vi "DrawTrail.vi"(8 "error in (no error)":errorcluster, 11 "Pong in":refnum<class "Pong.lvclass">) -> (0 "error out":errorcluster, 3 "Pong out":refnum<class "Pong.lvclass">)   [LabVIEW 2019, in "RT_Game.lvlib" / "Pong.lvclass"]
uses:
  Pong.lvclass
  Game/Coordinate.ctl
  Pong.lvclass/Pong.ctl
  PongBall/PongBall.lvclass
  C:/Users/FreshBob/Dropbox/VIs/myRIO_GameConsole/RT/RT_Game/GameObject/GameObject.lvclass
  Globals.vi
  GameObject/GameObject.lvclass
  Game/Game.lvclass
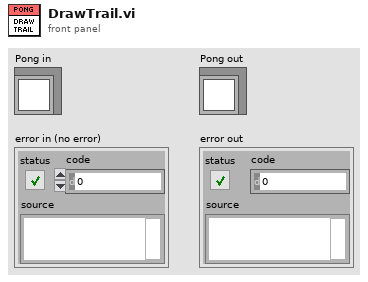
[diagram p1: front panel]
types:
  T1 = typedef "RT_Game.lvlib/Game.lvclass/Coordinate.ctl" = cluster{"x":dbl, "y":dbl}
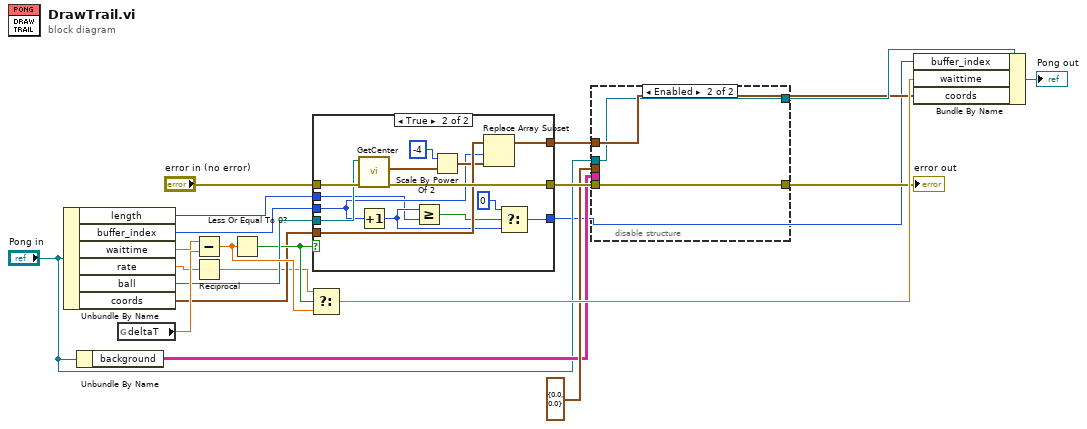
[diagram p0: block diagram]
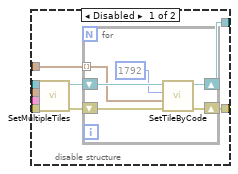
[diagram p2: hidden frame]
diagram:
  n1 = Unbundle By Name("Pong in") -> ("length"=w1:i16, "buffer_index"=w3:i16, "waittime"=w18:dbl, "rate"=w11:dbl, "ball"=w14:refnum<class "PongBall.lvclass">, "coords"=w12:T1[])
  n2 = Unbundle By Name("Pong in") -> ("background"=w5:string[][])
  n3 = global read "Globals.vi" "deltaT"() -> (w17:dbl)
  n4 = Subtract(x=w18, y=w17) -> (x-y=w16:dbl)
  n5 = Reciprocal(x=w11) -> (1/x=w10:dbl)
  n6 = Less Or Equal To 0?(x=w16) -> (x <= 0?=w13:bool)
  n7 = Select(t=w10, s=w13, f=w16) -> (s? t:f=w15:dbl)
  n8 = case shown="True" w13 {
    tunnel: [w24 w37] -> w20
    tunnel: "error in (no error)" -> [w24 w35]
    tunnel: w14 -> [_ w34]
    tunnel: w12 -> [w23 w33]
    tunnel: [w23 w32] -> w7
    tunnel: w3 -> [w22 w30]
    tunnel: [w22 w27] -> w2
    tunnel: w1 -> [_ w28]
    frame False {
    }
    frame True {
      n9 = call "GetCenter.vi"("error in (no error)"=w35, "GameObject in"=w34) -> ("error out"=w37:errorcluster, "center_pos"=w38:T1)  [unwired: 7 in, 1 out]
      n10 = Increment(x=w30) -> (x+1=w29:i16)
      n11 = Greater Or Equal?(x=w29, y=w28) -> (x >= y?=w26:bool)
      n12 = Scale By Power Of 2(n=i16 -4, x=w38) -> (x*2^n=w31:T1)
      n13 = Replace Array Subset(array=w33, new element=w31, index=w30) -> (w32:T1[])
      n14 = Select(t=i16 0, s=w26, f=w29) -> (s? t:f=w27:i16)
    }
  }
  n15 = disable-structure shown="Enabled" {
    disable-tunnel: w20 -> [w47 w55]
    disable-tunnel: [w46 w55] -> w9
    disable-tunnel: [w45 w54] -> w8
    disable-tunnel: w7 -> [w44 _]
    disable-tunnel: T1 {"x"=0.0, "y"=0.0} ("Position") -> [w41 _]
    disable-tunnel: w5 -> [w40 _]
    disable-tunnel: "Pong in" -> [w39 w54]
    frame Disabled {
      n16 = call "SetMultipleTiles.vi"("error in (no error)"=w47, "TileCodes"=w40, "Position"=w41, "Game in"=w39) -> ("error out"=w43:errorcluster, "Game out"=w42:refnum<class "Game.lvclass">)  [unwired: 6 in]
      n17 = for {
        shift-right: [w52] -> w46
        shift-left: w43 -> [w53]
        shift-right: [w50] -> w45
        shift-left: w42 -> [w51]
        tunnel: w44 -> [w49] mode=indexing
        n18 = call "SetTileByCode.vi"("error in (no error)"=w53, "Coordinates"=w49, "TileNumber"=u16 1792, "Game in"=w51) -> ("error out"=w52:errorcluster, "Game out"=w50:refnum<class "Game.lvclass">)  [unwired: 6 in]
      }
    }
    frame Enabled {
    }
  }
  "error out" <- w9
  n19 = Bundle By Name(cluster=w8, "buffer_index"=w2, "waittime"=w15, "coords"=w7) -> (→"Pong out":refnum<class "Pong.lvclass">)
